vi "WriteCDIndex.vi"(8 "error in (no error)":errorcluster, 10 "CDIndex":dbl, 11 "Stereo in":refnum<class "Stereo.lvclass">) -> (0 "error out":errorcluster, 3 "Stereo out":refnum<class "Stereo.lvclass">)   [LabVIEW 2013, in "Stereo.lvclass"]
uses:
  Stereo.lvclass
  Stereo.lvclass/Stereo.ctl
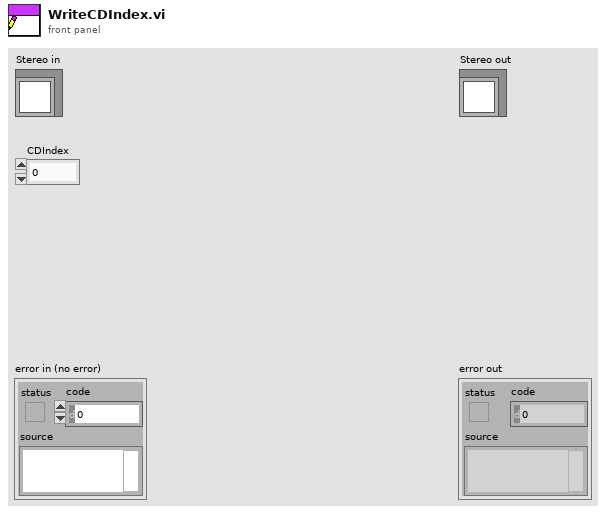
[diagram p1: front panel]
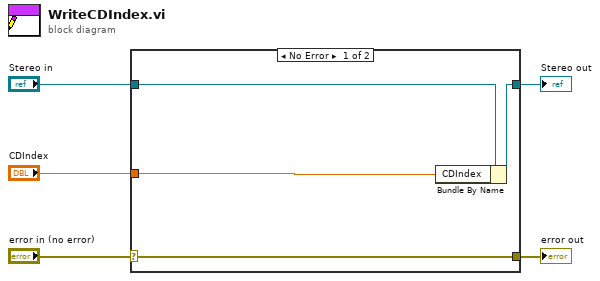
[diagram p0: block diagram]
diagram:
  n1 = case shown="No Error" "error in (no error)" {
    selector: "error in (no error)" -> [w9 w10]
    tunnel: [w9 w10] -> w4
    tunnel: [w7 w11] -> w2
    tunnel: "Stereo in" -> [w8 w11]
    tunnel: "CDIndex" -> [w6 _]
    frame No Error {
      n2 = Bundle By Name(cluster=w8, "CDIndex"=w6) -> (w7:refnum<class "Stereo.lvclass">)
    }
    frame Error {
    }
  }
  "error out" <- w4
  "Stereo out" <- w2
